vi "valve_control_output.vi"(1 "Voltages":dbl[](array[numeric]), 2 "Liquid channel":tag="cDAQ1Mod4/ao3", 3 "Vapor channel":tag="cDAQ1Mod4/ao2") -> ()   [LabVIEW 2015]
uses:
  <vilib>/DAQmx/create/channels.llb/DAQmx Create Channel (AO-Voltage-Basic).vi
  <vilib>/DAQmx/configure/timing.llb/DAQmx Timing (Sample Clock).vi
  <resource>/objmgr/daqmx.rc
  <vilib>/DAQmx/write.llb/DAQmx Write (Analog 1D Wfm NChan NSamp).vi
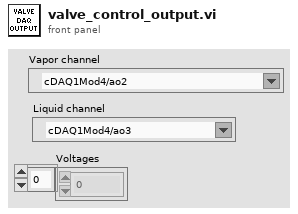
[diagram p1: front panel]
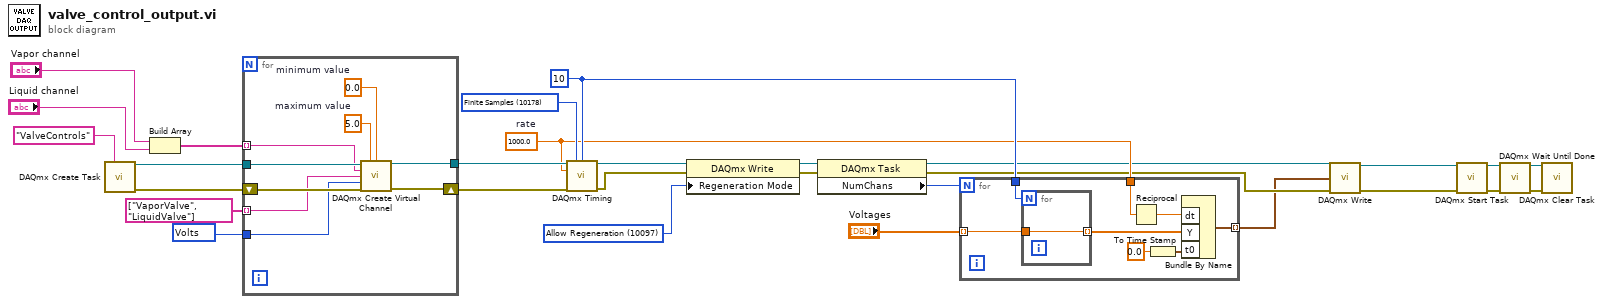
[diagram p0: block diagram]
diagram:
  w16 = 10097 items=["Allow Regeneration"=10097, "Do Not Allow Regeneration"=10158] ("RegenMode")
  w11 = 10 ("samples per channel")
  w19 = 10178 items=["Finite Samples"=10178, "Continuous Samples"=10123, "Hardware Timed Single Point"=12522] ("sample mode")
  w10 = 1000.0  # rate
  w25 = 10348 items=["Volts"=10348, "From Custom Scale"=10065] ("units")
  n1 = call <vilib>:"DAQmx Create Task.vi"("new task name"="ValveControls") -> ("task out"=w28:refnum<k21>, "error out"=w27:errorcluster)  [unwired: 13 in]
  n2 = Build Array("Vapor channel", "Liquid channel") -> (w22:tag[])
  n3 = for {
    tunnel: w28 -> [w38]
    shift-right: [w30] -> w20
    shift-left: w27 -> [w37]
    tunnel: string[] ["VaporValve", "LiquidValve"] -> [w36] mode=indexing
    tunnel: w25 -> [w35]
    tunnel: w22 -> [w34] mode=indexing
    tunnel: [w31] -> w21
    w32 = 0.0  # minimum value
    w33 = 5.0  # maximum value
    n4 = call-poly <vilib>:"DAQmx Create Virtual Channel.vi"("task in"=w38, "maximum value"=w33, "minimum value"=w32, "physical channels"=w34, "name to assign"=w36, "units"=w35, "error in"=w37) -> ("task out"=w31:refnum<k21>, "error out"=w30:errorcluster)  [unwired: 7 in]
  }
  n5 = call-poly <vilib>:"DAQmx Timing.vi"("task/channels in"=w21, "sample mode"=w19, "samples per channel"=w11, "rate"=w10, "error in"=w20) -> ("task out"=w18:refnum<k21>, "error out"=w17:errorcluster)  [unwired: 9 in]
  n6 = property class="DAQmx Write"(reference=w18, error in=w17, "Regeneration Mode"=w16) -> (reference out=w15:refnum<k21>, error out=w14:errorcluster)
  n7 = property class="DAQmx Task"(reference=w15, error in=w14) -> (reference out=w9:refnum<k21>, error out=w8:errorcluster, "NumChans"=w13:u32)
  n8 = for {
    N: w13 -> [_]
    tunnel: [w46] -> w7 mode=indexing
    tunnel: "Voltages" -> [w45] mode=indexing
    tunnel: w11 -> [w41]
    tunnel: w10 -> [w39]
    n9 = for {
      N: w41 -> [_]
      tunnel: w45 -> [w47]
      tunnel: [w47] -> w44 mode=indexing
    }
    n10 = Reciprocal(x=w39) -> (1/x=w40:dbl)
    n11 = To Time Stamp(1:0.0 ("number")) -> (0:w43:timestamp)
    n12 = Bundle By Name("dt"=w40, "Y"=w44, "t0"=w43) -> (w46:waveform(dbl))  [unwired: 1 out]
  }
  n13 = call-poly <vilib>:"DAQmx Write.vi"("task/channels in"=w9, "data"=w7, "error in"=w8) -> ("task out"=w6:refnum<k21>, "error out"=w5:errorcluster)  [unwired: 10 in, 1 out]
  n14 = call <vilib>:"DAQmx Start Task.vi"("task/channels in"=w6, "error in"=w5) -> ("task out"=w4:refnum<k21>, "error out"=w3:errorcluster)  [unwired: 12 in]
  n15 = call <vilib>:"DAQmx Wait Until Done.vi"("task/channels in"=w4, "error in"=w3) -> ("task out"=w2:refnum<k21>, "error out"=w1:errorcluster)  [unwired: 12 in]
  n16 = call <vilib>:"DAQmx Clear Task.vi"("task in"=w2, "error in"=w1) -> ()  [unwired: 13 in, 1 out]
